vi "_Ref To DVR.vi"(1 "TagDB":T1) -> (0 "DVR":refnum<data-value>)   [LabVIEW 2017, in "TagDB(DEV).lvlib"]
uses:
  TagDB(DEV).lvlib
  Typedef/TagDB.ctl
  Typedef/tagdb-data.ctl
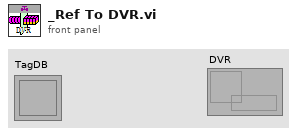
[diagram p1: front panel]
types:
  T1 = typedef "TagDB(DEV).lvlib/TagDB.ctl" = refnum<k1>
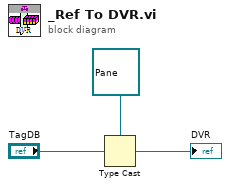
[diagram p0: block diagram]
diagram:
  n1 = Type Cast(type=refnum<data-value> refnum ("data value reference"), x="TagDB") -> (*(type *) &x=→"DVR":refnum<data-value>)
